vi "niDTS BT BDR Tx Test Get Default Parameters.vi"(0 "Dummy Test Handle In":T9, 11 "error in (no error)":errorcluster) -> (4 "Dummy Test Handle Out":T9, 8 "BDR Tx Parameters":T1={"Channel"=1, "Dut Tx Power (dBm)"=0.0, "Auto Level"=FALSE, "External Attenuation (dB)"=0.0, "BDR Packet type"=enum."DH1", "Payload Data"=enum."00001111", "Burst Sync"=enum."NONE", "Packet length (bytes)"=1500, "BD ADDRESS"="", "Modulation Measurement"={"ModAcc Enable"=FALSE, "CFO Enable"=FALSE, "Character Select"=enum."DF1", "Averages"=3, "Averaging Mode"=enum."RMS", "Measurement Duration (Symbols)"=0, "Measurement Offset (Symbols)"=0}, "Trace Enable"=FALSE, "OBW Measurement"={"OBW Enable"=FALSE, "OBW Averages"=3, "Averaging Type"=enum."RMS", "Measurement Interval Mode"=enum."AUTO", "Measurement Interval Length (sec)"=0.00015}, "TXP Measurement"={"TXP Power Enable"=FALSE, "TXP Averages"=3, "Averaging Type"=enum."RMS"}, "IBE Measurement"={"IBE Enable"=FALSE, "IBE Averages"=164, "Averaging Type"=enum."LOG", "Numbe of Channels"=12329017, "Channel Mode"=enum."Centered", "Measurement Interval Mode"=enum."MANUAL", "Measurement Interval Length (sec)"=1.0}, "Trigger"={"MinQuietTimeDuration (sec)"=0.0, "TriggerDelay (sec)"=0.0, "TriggerEdge"=enum."RISing", "TriggerSource"=enum."IMMediate", "TriggerThreshold (dB)"=0.0, "TriggerTimeout (sec)"=0.0}} {"Trigger"."MinQuietTimeDuration (sec)" format="%#_6p"}, 15 "error out":errorcluster)   [LabVIEW 2014, in "niDTS BT.lvlib"]
uses:
  niDTS BT.lvlib
  Tx Test/Includes/niDTS BT Tx Test INC Handle.ctl
  Tx Test/Objects/BASE_class/niDTS BT Tx Test.lvclass
  Includes/niDTS BT BDR Tx Test INC Parameters.ctl
  Includes/niDTS BT INC BDR Packet Type.ctl
  Tx Test/Includes/niDTS BT Tx Test INC BD Payload Data.ctl
  Tx Test/Includes/niDTS BT Tx Test INC Modulation Characteristics.ctl
  Includes/niDTS BT INC OBW Measurement Parameters.ctl
  Includes/niDTS BT INC TXP Measurement Parameters.ctl
  Includes/niDTS BT INC BDR ACP Measurement Parameters.ctl
  Includes/niDTS BT DUT INC Trigger.ctl
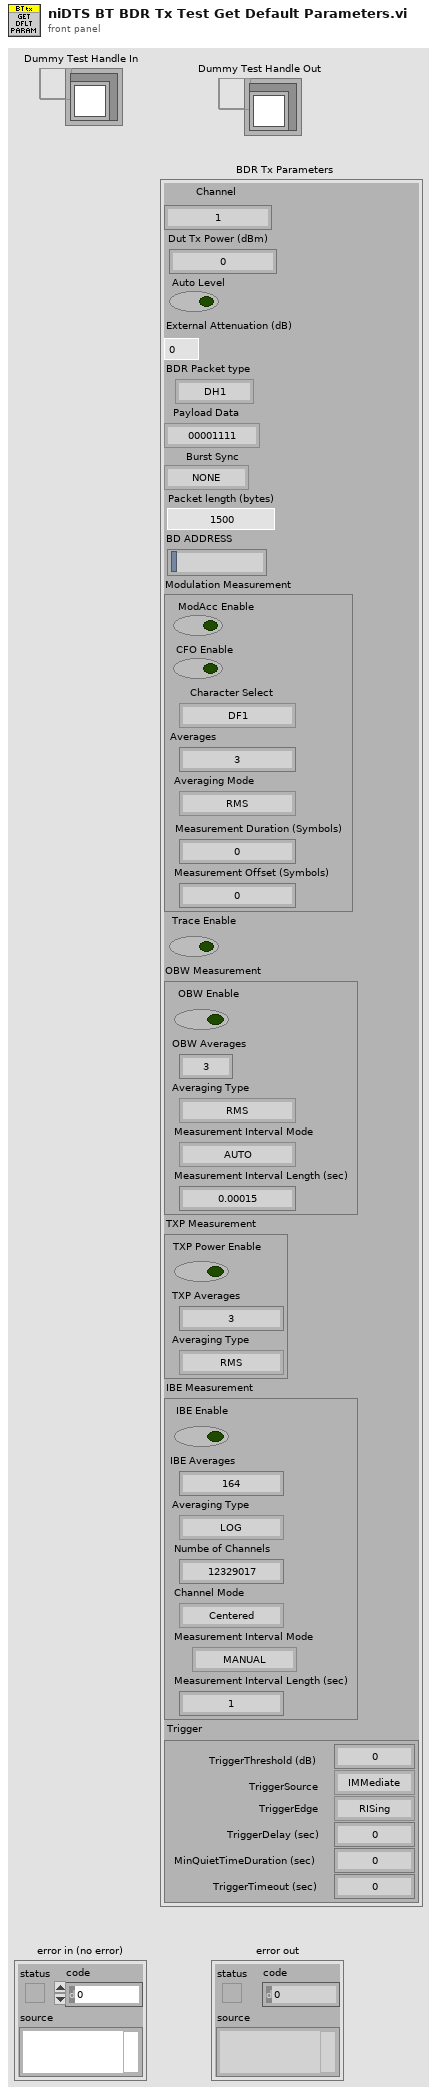
[diagram p1: front panel]
types:
  T1 = typedef "niDTS BT.lvlib/niDTS BT BDR Tx Test INC Parameters.ctl" = cluster{"Channel":i32, "Dut Tx Power (dBm)":dbl, "Auto Level":bool, "External Attenuation (dB)":dbl, "BDR Packet type":T2, "Payload Data":T3, "Burst Sync":enum16{"NONE", "PREamble"}, "Packet length (bytes)":i32, "BD ADDRESS":string, "Modulation Measurement":cluster{"ModAcc Enable":bool, "CFO Enable":bool, "Character Select":T4, "Averages":i32, "Averaging Mode":enum16{"RMS", "LOG", "SCALAR", "MAX", "MIN", "VECTOR"}, "Measurement Duration (Symbols)":i32, "Measurement Offset (Symbols)":i32}, "Trace Enable":bool, "OBW Measurement":T5, "TXP Measurement":T6, "IBE Measurement":T7, "Trigger":T8}
  T2 = typedef "niDTS BT.lvlib/niDTS BT INC BDR Packet Type.ctl" = enum16{"NULL", "POLL", "FHS", "DM1", "DH1", "HV1", "HV2", "HV3", "EV3", "DV", "AUX1", "DM3", "DH3", "EV4", "EV5", "DM5", "DH5"}
  T3 = typedef "niDTS BT.lvlib/niDTS BT Tx Test INC BD Payload Data.ctl" = enum16{"0", "1", "01", "00001111", "PN9", "AUTO"}
  T4 = typedef "niDTS BT.lvlib/niDTS BT Tx Test INC Modulation Characteristics.ctl" = enum16{"DF1", "DF2", "BOTH"}
  T5 = typedef "niDTS BT.lvlib/niDTS BT INC OBW Measurement Parameters.ctl" = cluster{"OBW Enable":bool, "OBW Averages":i32, "Averaging Type":enum16{"RMS", "LOG", "SCALAR", "MAX", "MIN", "VECTOR"}, "Measurement Interval Mode":enum16{"AUTO", "MANUAL"}, "Measurement Interval Length (sec)":dbl}
  T6 = typedef "niDTS BT.lvlib/niDTS BT INC TXP Measurement Parameters.ctl" = cluster{"TXP Power Enable":bool, "TXP Averages":i32, "Averaging Type":enum16{"RMS", "LOG", "SCALAR", "MAX", "MIN"}}
  T7 = typedef "niDTS BT.lvlib/niDTS BT INC BDR ACP Measurement Parameters.ctl" = cluster{"IBE Enable":bool, "IBE Averages":i32, "Averaging Type":enum16{"RMS", "LOG", "SCALAR", "MAX", "MIN", "VECTOR"}, "Numbe of Channels":i32, "Channel Mode":enum16{"InBand", "Centered"}, "Measurement Interval Mode":enum16{"AUTO", "MANUAL"}, "Measurement Interval Length (sec)":dbl}
  T8 = typedef "niDTS BT.lvlib/niDTS BT DUT INC Trigger.ctl" = cluster{"MinQuietTimeDuration (sec)":dbl, "TriggerDelay (sec)":dbl, "TriggerEdge":enum16{"RISing", "FALLing"}, "TriggerSource":enum16{"IMMediate", "RF0", "PFI0", "PFI1", "RTS0", "RTS1", "RTS2", "RTS3", "RTS4", "RTS5", "RTS6", "RTS7", "PXIStar", "SOFT"}, "TriggerThreshold (dB)":dbl, "TriggerTimeout (sec)":dbl}
  T9 = typedef "niDTS BT.lvlib/niDTS BT Tx Test INC Handle.ctl" = refnum<data-value>
  T10 = typedef "niDTS BT.lvlib/niDTS BT Tx Test INC Parameters.ctl" = cluster{"Channel":i32, "Data Rate ":i32, "Dut Tx Power":dbl, "External Attenuation (dB)":dbl[], "Auto Level":bool, "Packet type":T11, "Payload Pattern":T3, "Burst Sync":enum16{"NONE", "PREamble"}, "BD ADDRESS":u32, "Packet Length, bytes":i32, "ModAcc Measurement Paramaters":cluster{"ModAcc Enable":bool, "CFO Enable":bool, "Character Select":T12, "Averages":i32, "Averaging Mode":enum16{"RMS", "LOG", "SCALAR", "MAX", "MIN", "VECTOR"}, "Measurement Length":i32, "Measurement Offset":i32}, "OBW Measurement Parameters":T5, "TXP Measurement Parameters":T6, "IBE  Measurement Parameters":T13, "Trace Enable":bool, "Trigger":T8}
  T11 = typedef "niDTS BT.lvlib/niDTS BT INC Packet Type.ctl" = enum16{"NULL", "POLL", "FHS", "DM1", "DH1", "HV1", "HV2", "HV3", "EV3", "DV", "AUX1", "DM3", "DH3", "EV4", "EV5", "DM5", "DH5", "LE-TP"}
  T12 = typedef "niDTS BT Tx Test INC Modulation Characteristics.ctl" = enum16{"DF1", "DF2", "BOTH"}
  T13 = typedef "niDTS BT.lvlib/niDTS BT INC EDR IBE Measurement Parameters.ctl" = cluster{"IBE Enable":bool, "IBE Averages":i32, "Averaging Type":enum16{"RMS", "LOG", "SCALAR", "MAX", "MIN", "VECTOR"}, "Numbe of Channels":i32, "Channel Mode":enum16{"InBand", "Centered"}, "Measurement Interval Mode":enum16{"AUTO", "MANUAL"}, "Measurement Interval Length (sec)":dbl}
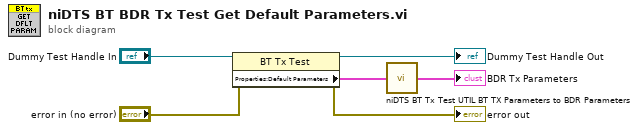
[diagram p0: block diagram]
diagram:
  n1 = property class="BT Tx Test"(reference="Dummy Test Handle In", error in="error in (no error)") -> (reference out=→"Dummy Test Handle Out":T9, error out=→"error out":errorcluster, "Properties:Default Parameters"=w2:T10)
  n2 = call "niDTS BT Tx Test UTIL BT TX Parameters to BDR Parameters.vi"("Default Parameters"=w2) -> ("output cluster"=→"BDR Tx Parameters":T1)  [unwired: 14 in]
